vi "Proyecto_final.vi"() -> ()   [LabVIEW 2020]
uses:
  <vilib>/Instr/_visa.llb/VISA Configure Serial Port (Instr).vi
panel:
  out "read buffer":string
  in  "VISA resource name":refnum<visa-resource-name>
  out "Hora":string
  out "Fecha":string
  in  "Hora":bool
  in  "Fecha":bool
  in  "Dosis":dbl(knob) scale=100.0..200.0
  in  "Medicamento":bool
  out "Gráfica de flujo vs Tiempo":i32(graph)
  out "Flujo_Emitido":string
  in  "Graficar":bool
  in  "stop":bool
  # "Medición de flujo"
  # "Graficar"
  # "Dosis de medicamentos"
  # "Fecha y hora"
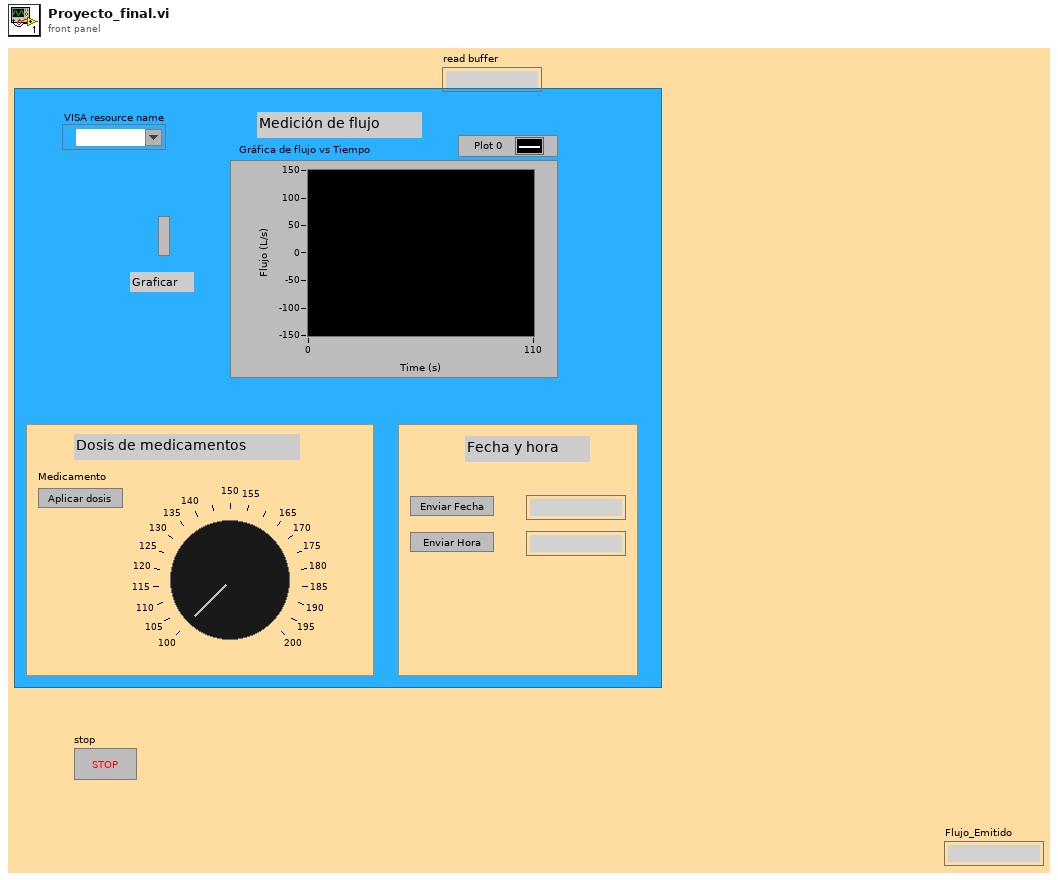
[diagram p1: front panel]
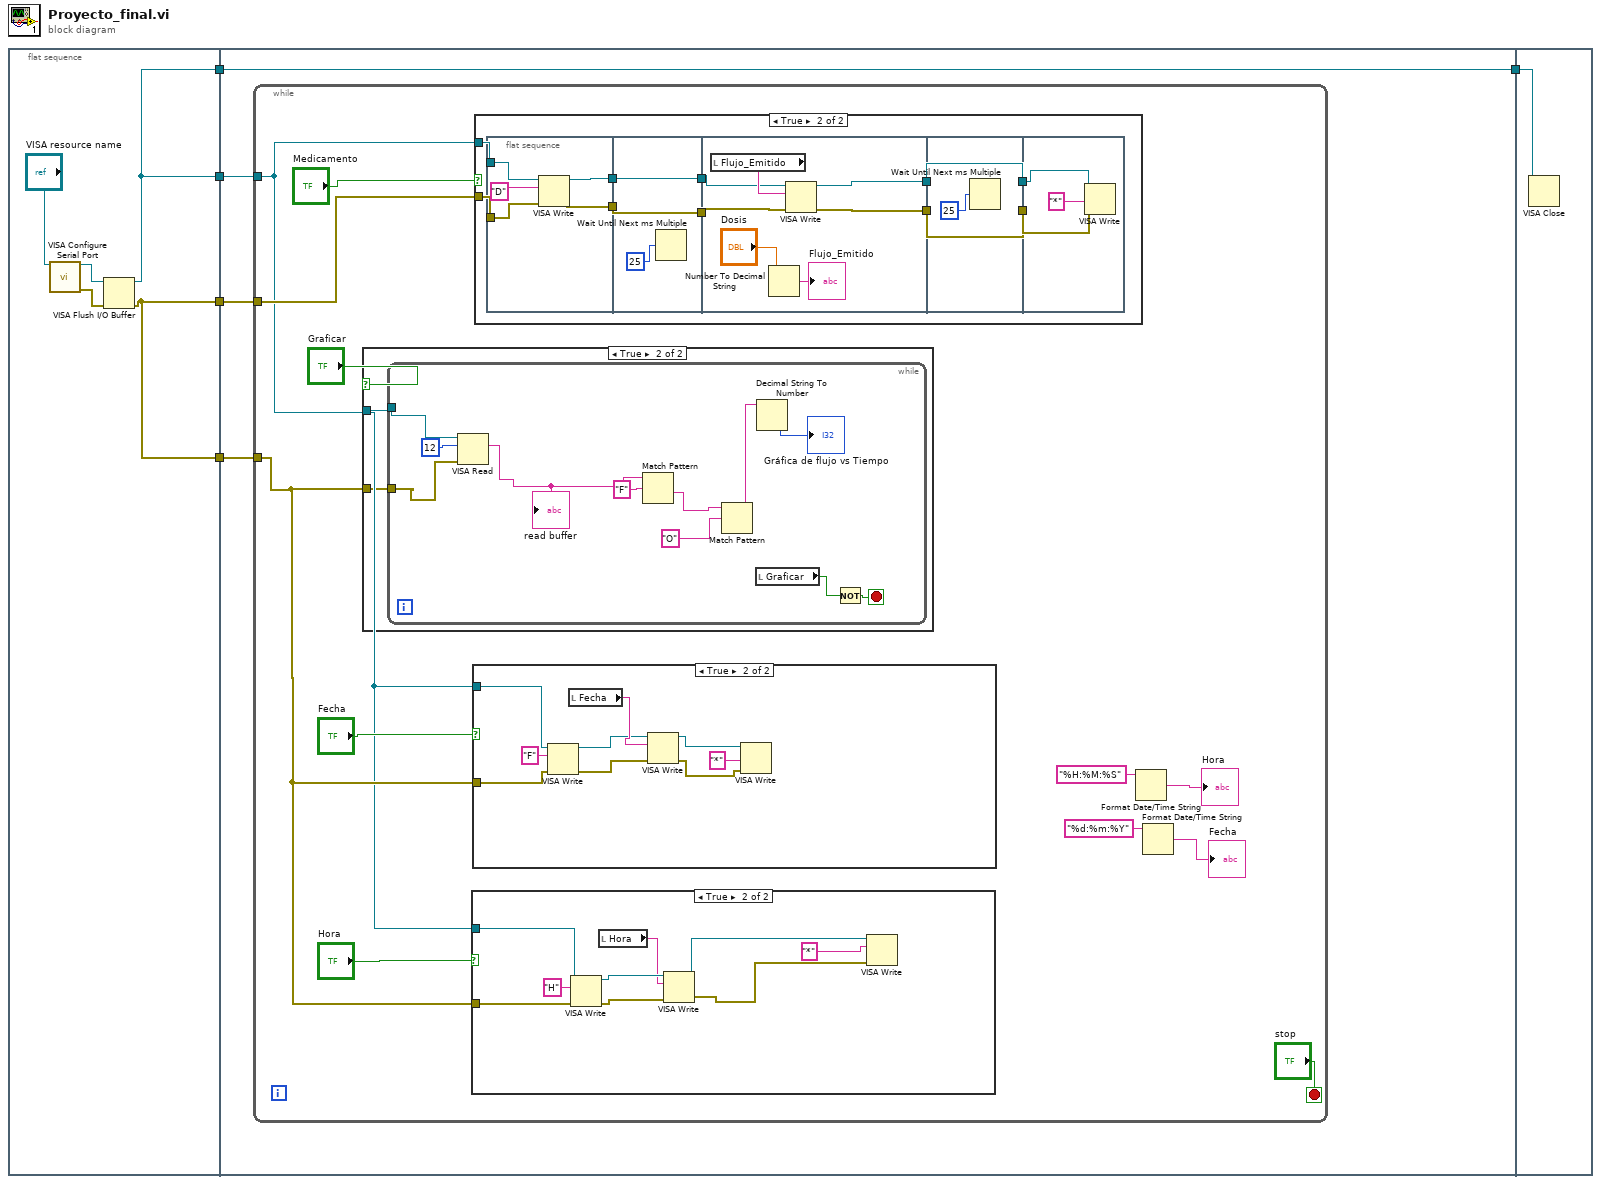
[diagram p0: block diagram]
diagram:
  n1 = flat-sequence {
    tunnel: [w8] -> w5
    tunnel: [w8] -> w3
    tunnel: [w7] -> w2
    tunnel: [w7] -> w1
    tunnel: w5 -> [w14]
    tunnel: [w14] -> w4
    tunnel: w3 -> [w13]
    tunnel: w2 -> [w12]
    tunnel: w1 -> [w11]
    tunnel: w4 -> [w89]
    frame #0 {
      n2 = call-poly "VISA Configure Serial Port"("VISA resource name"="VISA resource name") -> ("VISA resource name out"=w10:refnum<visa-resource-name>, "error out"=w9:errorcluster)  [unwired: 13 in]
      n3 = VISA Flush I/O Buffer(VISA resource name=w10, error in (no error)=w9) -> (VISA resource name out=w8:refnum<visa-resource-name>, error out=w7:errorcluster)  [unwired: 1 in]
    }
    frame #1 {
      n4 = while {
        tunnel: w13 -> [w15]
        tunnel: w12 -> [w16]
        tunnel: w11 -> [w23]
        stop <- "stop" stop-if-true
        n5 = case shown="True" "Graficar" {
          tunnel: w16 -> [_ w76]
          tunnel: w15 -> [_ w77]
          frame False {
          }
          frame True {
            n6 = while {
              tunnel: w77 -> [w88]
              tunnel: w76 -> [w87]
              stop <- w81 stop-if-true
              n7 = VISA Read(VISA resource name=w88, byte count=u32 12, error in (no error)=w87) -> (read buffer=w86:string)  [unwired: 3 out]
              "read buffer" <- w86
              n8 = Match Pattern(string=w86, regular expression="F") -> (after substring=w82:string)  [unwired: 1 in, 3 out]
              n9 = Match Pattern(string=w82, regular expression="O") -> (before substring=w79:string)  [unwired: 1 in, 3 out]
              n10 = local read "Graficar"() -> (w80:bool)
              n11 = Decimal String To Number(string=w79) -> (number=→"Gráfica de flujo vs Tiempo":i32)  [unwired: 2 in, 1 out]
              n12 = Not(x=w80) -> (.not. x?=w81:bool)
            }
          }
        }
        n13 = case shown="True" "Hora" {
          tunnel: w16 -> [_ w34]
          tunnel: w15 -> [_ w33]
          frame False {
          }
          frame True {
            n14 = VISA Write(VISA resource name=w33, write buffer="H", error in (no error)=w34) -> (VISA resource name out=w32:refnum<visa-resource-name>, error out=w31:errorcluster)  [unwired: 1 out]
            n15 = local read "Hora"() -> (w30:string)
            n16 = VISA Write(VISA resource name=w32, write buffer=w30, error in (no error)=w31) -> (VISA resource name out=w29:refnum<visa-resource-name>, error out=w28:errorcluster)  [unwired: 1 out]
            n17 = VISA Write(VISA resource name=w29, write buffer="*", error in (no error)=w28) -> ()  [unwired: 3 out]
          }
        }
        n18 = case shown="True" "Fecha" {
          tunnel: w15 -> [_ w43]
          tunnel: w16 -> [_ w42]
          frame False {
          }
          frame True {
            n19 = VISA Write(VISA resource name=w43, write buffer="F", error in (no error)=w42) -> (VISA resource name out=w40:refnum<visa-resource-name>, error out=w39:errorcluster)  [unwired: 1 out]
            n20 = local read "Fecha"() -> (w41:string)
            n21 = VISA Write(VISA resource name=w40, write buffer=w41, error in (no error)=w39) -> (VISA resource name out=w36:refnum<visa-resource-name>, error out=w37:errorcluster)  [unwired: 1 out]
            n22 = VISA Write(VISA resource name=w36, write buffer="*", error in (no error)=w37) -> ()  [unwired: 3 out]
          }
        }
        n23 = case shown="True" "Medicamento" {
          tunnel: w15 -> [_ w53]
          tunnel: w23 -> [_ w54]
          frame False {
          }
          frame True {
            n24 = flat-sequence {
              tunnel: w53 -> [w58]
              tunnel: w54 -> [w59]
              tunnel: [w56] -> w52
              tunnel: [w55] -> w50
              tunnel: w52 -> [w62]
              tunnel: [w62] -> w51
              tunnel: w50 -> [w61]
              tunnel: [w61] -> w49
              tunnel: w51 -> [w66]
              tunnel: w49 -> [w65]
              tunnel: [w64] -> w48
              tunnel: [w63] -> w47
              tunnel: w48 -> [w72]
              tunnel: w47 -> [w71]
              tunnel: [w72] -> w46
              tunnel: [w71] -> w45
              tunnel: w46 -> [w75]
              tunnel: w45 -> [w74]
              frame #0 {
                n25 = VISA Write(VISA resource name=w58, write buffer="D", error in (no error)=w59) -> (VISA resource name out=w55:refnum<visa-resource-name>, error out=w56:errorcluster)  [unwired: 1 out]
              }
              frame #1 {
                n26 = Wait Until Next ms Multiple(millisecond multiple=u32 25) -> ()  [unwired: 1 out]
              }
              frame #2 {
                n27 = local read "Flujo_Emitido"() -> (w69:string)
                n28 = Number To Decimal String(number="Dosis") -> (decimal integer string=→"Flujo_Emitido":string)  [unwired: 1 in]
                n29 = VISA Write(VISA resource name=w65, write buffer=w69, error in (no error)=w66) -> (VISA resource name out=w63:refnum<visa-resource-name>, error out=w64:errorcluster)  [unwired: 1 out]
              }
              frame #3 {
                n30 = Wait Until Next ms Multiple(millisecond multiple=u32 25) -> ()  [unwired: 1 out]
              }
              frame #4 {
                n31 = VISA Write(VISA resource name=w74, write buffer="*", error in (no error)=w75) -> ()  [unwired: 3 out]
              }
            }
          }
        }
        n32 = Format Date/Time String(time format string (%c)="%H:%M:%S") -> (date/time string=→"Hora":string)  [unwired: 2 in]
        n33 = Format Date/Time String(time format string (%c)="%d:%m:%Y") -> (date/time string=→"Fecha":string)  [unwired: 2 in]
      }
    }
    frame #2 {
      n34 = VISA Close(VISA resource name=w89) -> ()  [unwired: 1 in, 1 out]
    }
  }
